vi "WriteErrorDetails.vi"(8 "error in (no error)":errorcluster, 10 "ErrorDetails":T1[](array[typedef]), 11 "LabErrorUX in":refnum<class "LabErrorUX.lvclass">) -> (0 "error out":errorcluster, 3 "LabErrorUX out":refnum<class "LabErrorUX.lvclass">)   [LabVIEW 2019, in "LabErrorUX.lvclass"]
uses:
  LabErrorUX.lvclass
  LabErrorUX.lvclass/LabErrorUX.ctl
  Typedefs/ErrorUX.ctl
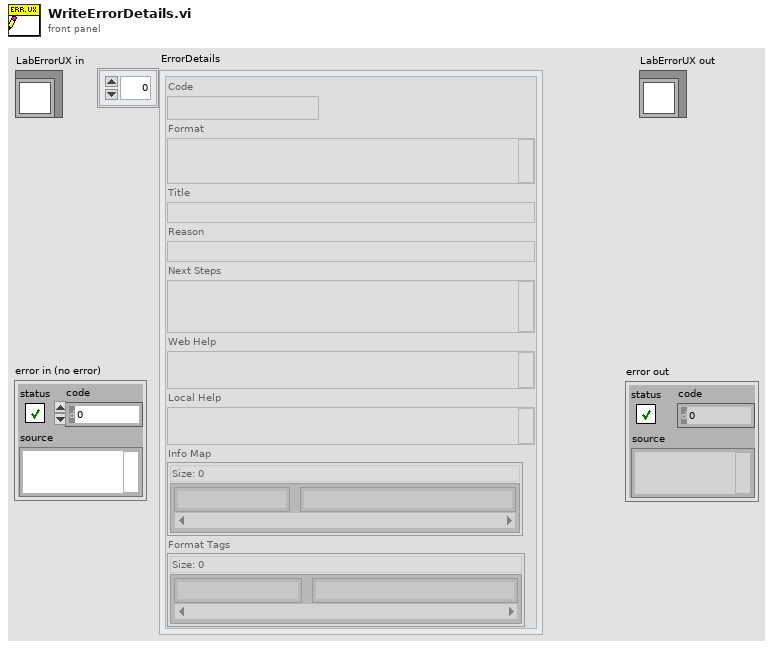
[diagram p1: front panel]
types:
  T1 = typedef "LabErrorUX.lvclass/ErrorUX.ctl" = cluster{"Code":string, "Format":string, "Title":string, "Reason":string, "Next Steps":string, "Web Help":string, "Local Help":string, "Info Map":map{string, string}, "Format Tags":map{string, string}}
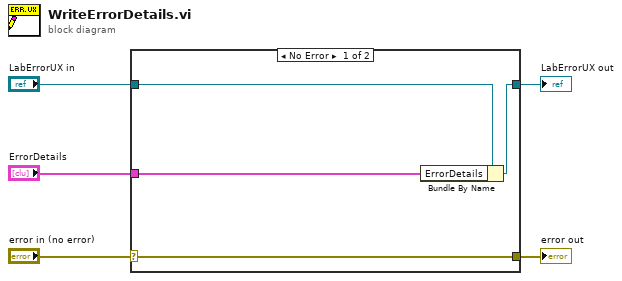
[diagram p0: block diagram]
diagram:
  n1 = case shown="No Error" "error in (no error)" {
    selector: "error in (no error)" -> [w9 w10]
    tunnel: [w9 w10] -> w4
    tunnel: [w7 w11] -> w2
    tunnel: "LabErrorUX in" -> [w8 w11]
    tunnel: "ErrorDetails" -> [w6 _]
    frame No Error {
      n2 = Bundle By Name(cluster=w8, "ErrorDetails"=w6) -> (w7:refnum<class "LabErrorUX.lvclass">)
    }
    frame Error {
    }
  }
  "error out" <- w4
  "LabErrorUX out" <- w2
